vi "TestPointer.Allocate Random Byte Array.vi"(8 "error in (no error)":errorcluster, 11 "Test Pointer in":refnum<class "TestPointer.lvclass">) -> (0 "error out":errorcluster, 3 "Test Pointer out":refnum<class "TestPointer.lvclass">)   [LabVIEW 2016, in "TestPointer.lvclass"]
uses:
  TestPointer.lvclass
panel:
  out "random byte array":u8[](array[numeric])
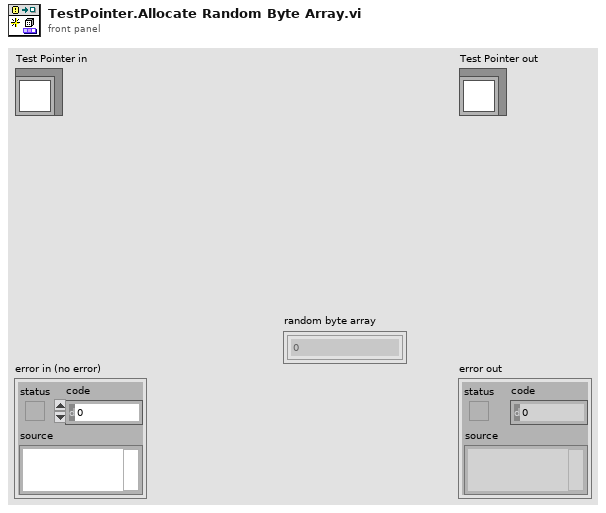
[diagram p1: front panel]
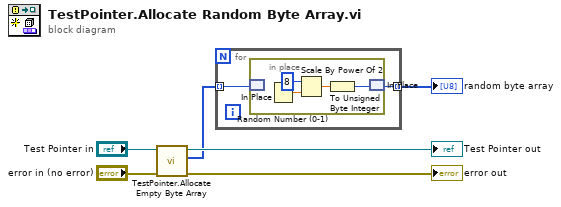
[diagram p0: block diagram]
diagram:
  n1 = call "TestPointer.Allocate Empty Byte Array.vi"("error in (no error)"="error in (no error)", "Test Pointer in"="Test Pointer in") -> ("error out"=→"error out":errorcluster, "empty byte array"=w1:u8[], "Test Pointer out"=→"Test Pointer out":refnum<class "TestPointer.lvclass">)  [unwired: 7 in]
  n2 = for {
    tunnel: w1 -> [w8] mode=indexing
    tunnel: [w7] -> w6 mode=indexing
    n3 = in-place {
      n4 = in-place-match #1(w8) -> ()  [unwired: 1 out]
      n5 = Random Number (0-1)() -> (number: 0 to 1=w10:dbl)
      n6 = Scale By Power Of 2(n=i16 8, x=w10) -> (x*2^n=w12:dbl)
      n7 = To Unsigned Byte Integer(number=w12) -> (unsigned 8bit integer=w9:u8)
      n8 = in-place-match #1(w9) -> (w7:u8)
    }
  }
  "random byte array" <- w6
